vi "通信状态入队列.vi"(8 "错误输入（无错误）":errorcluster, 11 "枚举":enum16{"打开连接", "发送数据", "读取数据", "数据处理", "关闭连接"}(ring)) -> (0 "错误输出":errorcluster)   [LabVIEW 2016, in "数据传输系统.lvlib"]
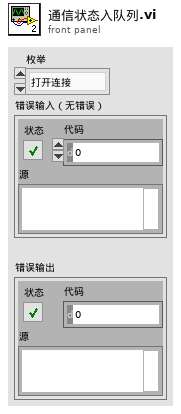
[diagram p1: front panel]
types:
  T1 = cluster{"setini":string, "sysini":string, "hechaini":string, "actualwrite":string, "actualread":string, "datasent":string, "反控命令信息队列":string, "反控与仪器交互":string}
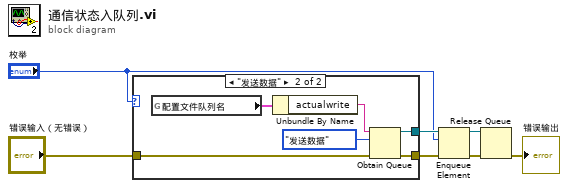
[diagram p0: block diagram]
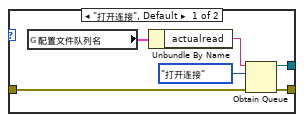
[diagram p2: hidden frame]
diagram:
  n1 = case shown="\"发送数据\"" "枚举" {
    tunnel: [w12 w18] -> w6
    tunnel: [w11 w17] -> w5
    tunnel: "错误输入（无错误）" -> [w10 w16]
    frame "打开连接", Default {
      n2 = global read "断电保存全局.vi" "配置文件队列名"() -> (w9:T1)
      n3 = Unbundle By Name(w9) -> ("actualread"=w8:string)
      n4 = Obtain Queue(name (unnamed)=w8, element data type=enum16{"打开连接", "发送数据", "读取数据", "数据处理", "关闭连接"}."打开连接" ("枚举"), error in (no error)=w10) -> (queue out=w12:refnum<queue>, error out=w11:errorcluster)  [unwired: 2 in, 1 out]
    }
    frame "发送数据" {
      n5 = global read "断电保存全局.vi" "配置文件队列名"() -> (w15:T1)
      n6 = Unbundle By Name(w15) -> ("actualwrite"=w14:string)
      n7 = Obtain Queue(name (unnamed)=w14, element data type=enum16{"打开连接", "发送数据", "读取数据", "数据处理", "关闭连接"}."发送数据" ("枚举"), error in (no error)=w16) -> (queue out=w18:refnum<queue>, error out=w17:errorcluster)  [unwired: 2 in, 1 out]
    }
  }
  n8 = Enqueue Element(queue=w6, element="枚举", error in (no error)=w5) -> (queue out=w7:refnum<queue>, error out=w4:errorcluster)  [unwired: 1 in, 1 out]
  n9 = Release Queue(queue=w7, error in (no error)=w4) -> (error out=→"错误输出":errorcluster)  [unwired: 1 in, 2 out]
